vi "errorexample.vi"() -> ()   [LabVIEW 2015]
panel:
  out "String":string="HAS TERMINADO"
  out "Cuadrado":i16=169
  out "Dato despues de encender el dispositivo":i32=7
  out "Dato antes de encender el dispositivo":dbl=4.9605129807700665
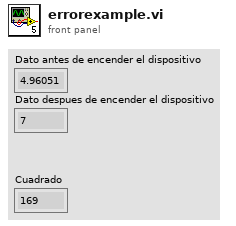
[diagram p1: front panel]
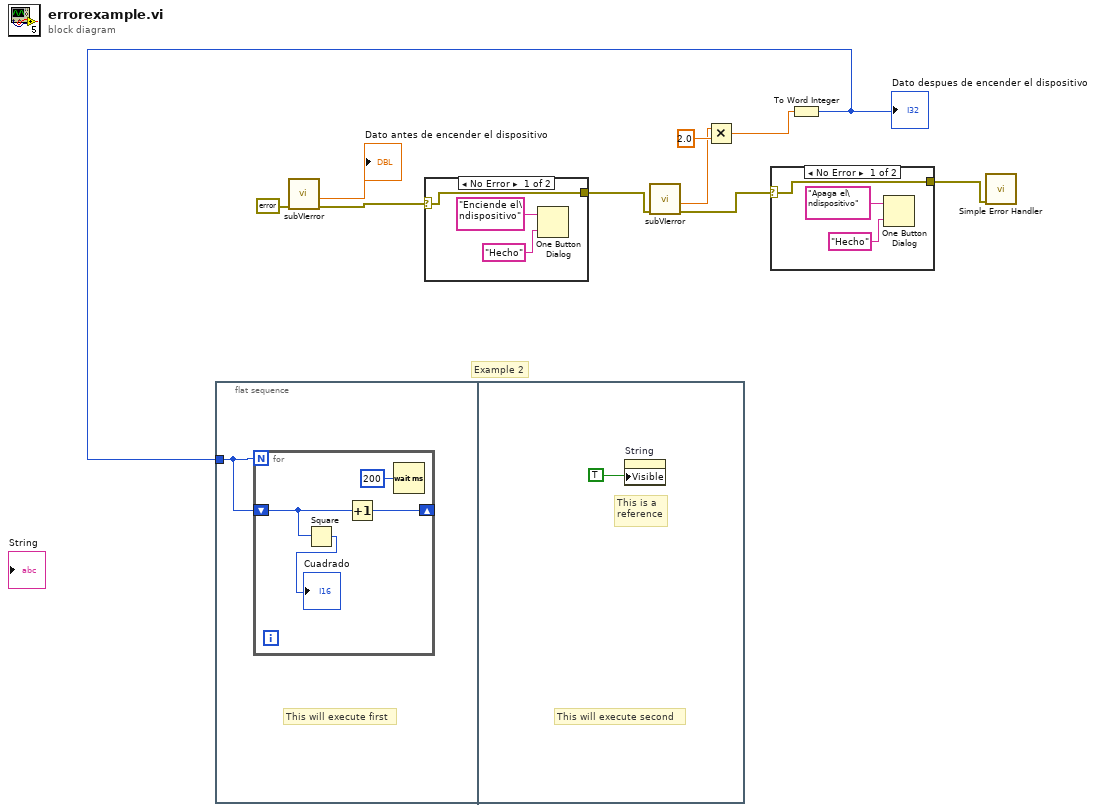
[diagram p0: block diagram]
diagram:
  # "Example 2"
  n1 = flat-sequence {
    tunnel: w1 -> [w11]
    frame #0 {
      # "This will execute first"
      n2 = for {
        N: w11 -> [_]
        shift-right: [w14] -> _
        shift-left: w11 -> [w13]
        n3 = Square(x=w13) -> (x^2=→"Cuadrado":i16)
        n4 = Increment(x=w13) -> (x+1=w14:i16)
        n5 = Wait (ms)(milliseconds to wait=u32 200) -> ()  [unwired: 1 out]
      }
    }
    frame #1 {
      # "This is a\nreference"
      # "This will execute second"
      n6 = property on="String" class="Str"("Visible"=TRUE) -> ()  [unwired: 2 in, 2 out]
    }
  }
  n7 = call "subVIerror.vi"("first error"=errorcluster {"status"=FALSE, "code"=0, "source"=""}) -> ("second \nerror"=w9:errorcluster, "x*y"=→"Dato antes de encender el dispositivo":dbl)  [unwired: 9 in]
  n8 = case shown="No Error" w9 {
    selector: w9 -> [w17 w20]
    tunnel: [w17 w20] -> w7
    frame No Error {
      n9 = One Button Dialog(message="Enciende el\ndispositivo", button name ("OK")="Hecho") -> ()  [unwired: 1 out]
    }
    frame Error {
    }
  }
  n10 = call "subVIerror.vi"("first error"=w7) -> ("second \nerror"=w10:errorcluster, "x*y"=w3:dbl)  [unwired: 9 in]
  n11 = Multiply(x=w3, y=2.0) -> (x*y=w2:dbl)
  n12 = case shown="No Error" w10 {
    selector: w10 -> [w21 w24]
    tunnel: [w21 w24] -> w6
    frame No Error {
      n13 = One Button Dialog(message="Apaga el\ndispositivo", button name ("OK")="Hecho") -> ()  [unwired: 1 out]
    }
    frame Error {
    }
  }
  n14 = To Word Integer(number=w2) -> (16bit integer=w1:i16)
  "Dato despues de encender el dispositivo" <- w1
  n15 = call <vilib>:"Simple Error Handler.vi"("error in (no error)"=w6) -> ()  [unwired: 4 in, 5 out]
